vi "Yscaling.vi"(8 "Nano Z Read":dbl, 9 "Current Maxed?":bool, 10 "Y":dbl, 11 "Plane Height":dbl) -> (3 "y scaled":dbl, 4 "Testoutput":dbl)   [LabVIEW 2017]
uses:
  <userlib>/HapticSTM/Feedbackless - Testdata/HapticSTM_Feedblackless_testdata Folder/HapticSTM.lvlib
panel:
  out "x*y":dbl
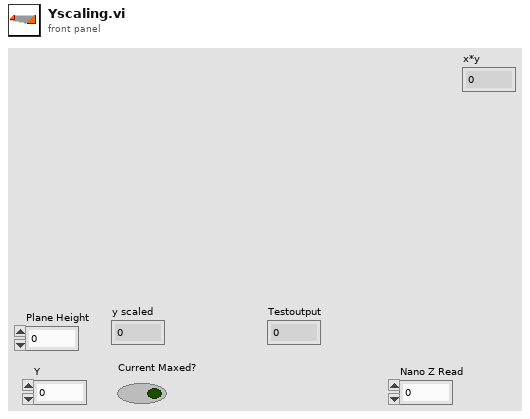
[diagram p1: front panel]
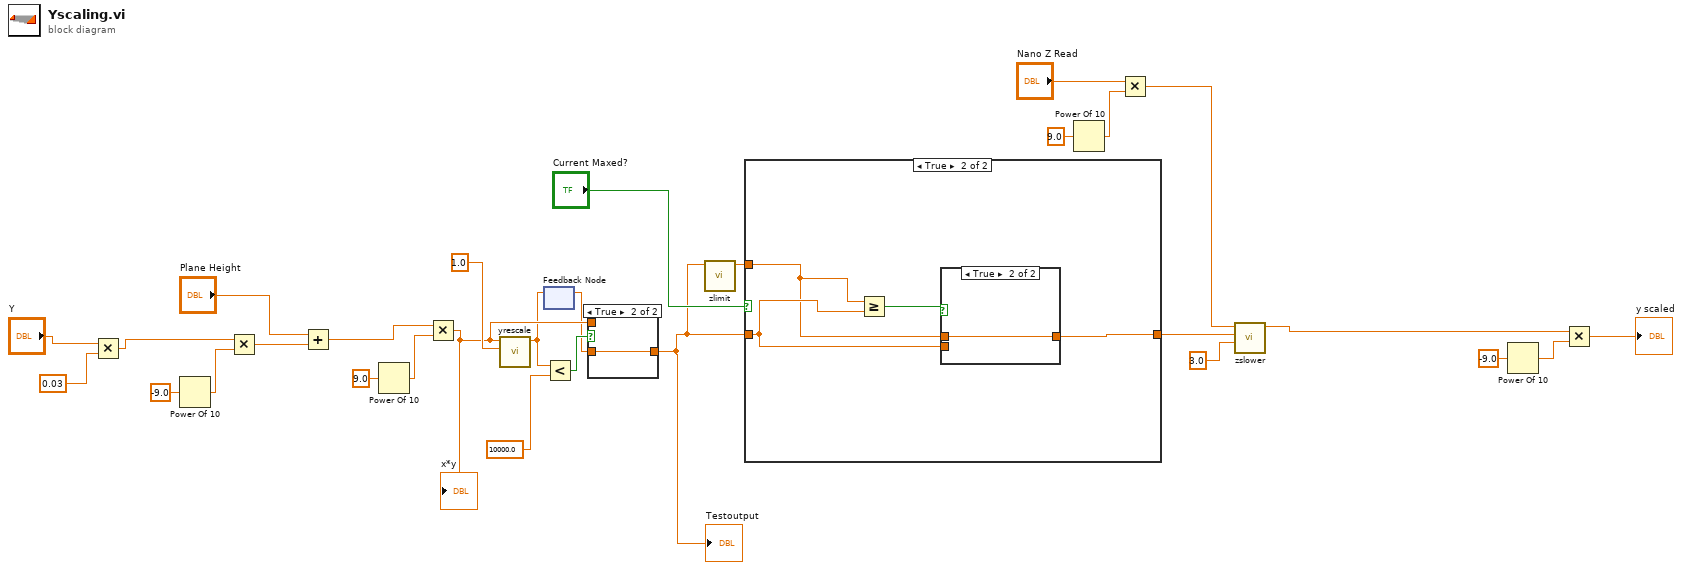
[diagram p0: block diagram]
diagram:
  n1 = Multiply(x="Y", y=0.03) -> (x*y=w25:dbl)
  n2 = Power Of 10(x=-9.0) -> (10^x=w24:dbl)
  n3 = Multiply(x=w25, y=w24) -> (x*y=w26:dbl)
  n4 = Add(x="Plane Height", y=w26) -> (x+y=w29:dbl)
  n5 = Power Of 10(x=9.0) -> (10^x=w28:dbl)
  n6 = Multiply(x=w29, y=w28) -> (x*y=w10:dbl)
  "x*y" <- w10
  n7 = call <userlib>:"yrescale.vi"("scalingfactor"=1.0, "ylabview"=w10) -> ("function return"=w9:dbl)  [unwired: 9 in]
  n8 = feedback-in #1(w9) -> ()
  n9 = feedback #1() -> (w8:dbl)  [unwired: 1 in]
  n10 = Less?(x=w9, y=10000.0) -> (x < y?=w11:bool)
  n11 = case shown="True" w11 {
    tunnel: [w30 w31] -> w13
    tunnel: w8 -> [_ w31]
    tunnel: w10 -> [w30 _]
    frame False {
    }
    frame True {
    }
  }
  "Testoutput" <- w13
  n12 = call <userlib>:"zlimit.vi"("yscaledinput"=w13) -> ("function return"=w14:dbl)  [unwired: 10 in]
  n13 = case shown="True" "Current Maxed?" {
    tunnel: [w32 w36] -> w7
    tunnel: w13 -> [w32 w34]
    tunnel: w14 -> [_ w33]
    frame False {
    }
    frame True {
      n14 = Greater Or Equal?(x=w33, y=w34) -> (x >= y?=w35:bool)
      n15 = case shown="True" w35 {
        tunnel: w33 -> [_ w38]
        tunnel: [w37 w38] -> w36
        tunnel: w34 -> [w37 _]
        frame False {
        }
        frame True {
        }
      }
    }
  }
  n16 = Power Of 10(x=9.0) -> (10^x=w4:dbl)
  n17 = Multiply(x="Nano Z Read", y=w4) -> (x*y=w1:dbl)
  n18 = call <userlib>:"zslower.vi"("maxvel"=3.0, "labview_zpos_write"=w7, "nanonis_zpos_read"=w1) -> ("function return"=w5:dbl)  [unwired: 8 in]
  n19 = Power Of 10(x=-9.0) -> (10^x=w17:dbl)
  n20 = Multiply(x=w5, y=w17) -> (x*y=→"y scaled":dbl)
